vi "Get Waveform.vi"(8 "error in (no error)":errorcluster, 10 "Save data":bool, 11 "Tektronix Driver in":refnum<class "Tektronix Driver.lvclass">) -> (0 "error out":errorcluster, 2 "Waveform":waveform(dbl), 3 "Tektronix Driver out":refnum<class "Tektronix Driver.lvclass">)   [LabVIEW 2020, in "Tektronix Driver.lvclass"]
uses:
  Tektronix Driver.lvclass
  Tektronix Driver.lvclass/Tektronix Driver.ctl
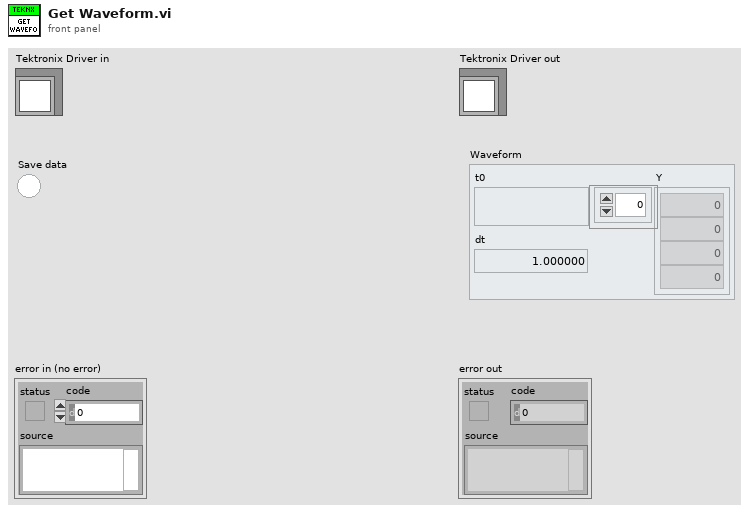
[diagram p1: front panel]
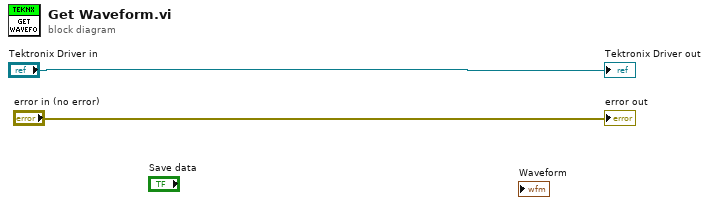
[diagram p0: block diagram]
diagram:
  "error out" <- "error in (no error)"
  "Tektronix Driver out" <- "Tektronix Driver in"
